vi "_io_viRead.vi"(8 "error in":errorcluster caption="error in (no error)", 9 "Allow Assure End with LF":bool=TRUE, 10 "Max bytes to read":u32=2048, 11 "VISA resource name":refnum<visa-resource-name>) -> (0 "error out":errorcluster, 1 "Read bytes count":u32, 2 "Read buffer":string, 3 "VISA resource name out":refnum<visa-resource-name>)   [LabVIEW 2020, in "Rohde&Schwarz RTx Oscilloscopes.lvlib" / "rsidr_core.lvlib"]
doc: "same as VISA viRead, but has an option to read the second time if the string was not ended with LF character"
uses:
  rsidr_core.lvlib
  type_AdditionalFlag_Bits.ctl
  type_Error_Codes.ctl
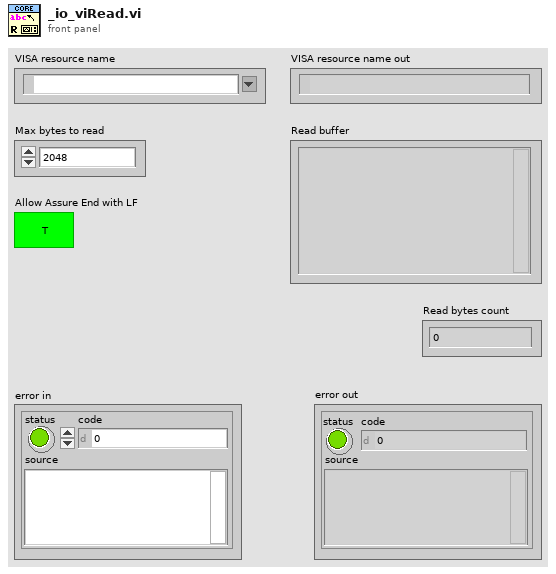
[diagram p1: front panel]
types:
  T1 = typedef "Rohde&Schwarz RTx Oscilloscopes.lvlib/rsidr_core.lvlib/type_AdditionalFlag_Bits.ctl" = enum16{"Send LF after Bin Block", "Junk read with io_clear_buffers.vi", "io_clear_buffers: viClear()", "io_clear_buffers: viFlush()", "<NotUsed1>", "Allow Dbl & Int Bin/Ascii read", "*OPC? in check_instrument_error.vi", "<NotUsed2>", "Smart Enum Matching", "Less Strict RepCaps check", "AssureResponseEndWithLF"}
  T2 = typedef "Rohde&Schwarz RTx Oscilloscopes.lvlib/rsidr_core.lvlib/type_Error_Codes.ctl" = enum16{"No_error", "VISA_err_ResourceNotFound", "VISA_err_Timeout", "VISA_warn_MoreDataAvailable", "RS_err_MissingCallback", "RS_err_InvalidAttribute", "RS_err_InvalidValue", "RS_err_UnknownResource", "RS_err_AlreadyInitialized", "RS_err_InstrumentStatus", "RS_err_BadRepCapName", "RS_err_TypesMismatch", "RS_err_ValueNotSupported", "RS_err_InvalidRngTable", "RS_err_IDqueryFail", "RS_err_UnexpResponse", "VISA_warn_ConfigNotLoaded", "RS_err_AttributeNotReadable", "RS_err_AttributeNotWritable", "RS_err_InstrumentType", "RS_err_InstrumentOption", "VISA_err_InvalidSize", "RS_err_ReliabilityIndicator", "VISA_warn_UnknownStatus", "VISA_warn_TermCharRead", "VISA_err_IO_error", "RS_err_FunctionNotSupported", "VISA_warn_QueueEmpty"}
  T3 = typedef "Rohde&Schwarz RTx Oscilloscopes.lvlib/rsidr_core.lvlib/type_Session_Data.ctl" = cluster{"IDN string":string, "Instrument FW":string, "Instr type":string, "Instr type for err. msg.":string, "Installed Options":string[], "Ignore Error Messages":string, "Logging params":variant, "OPC Timeout":i32, "VISA Timeout":i32, "STB Poll VISA Timeout":i32, "Additional Flags":i32, "Wait Before Read":i32, "Wait Before Write":i32, "Option String Flags":i32, "IO Segment Size":i64, "VISA Access Mode":T4, "Interface Type":T5, "OPC Wait Mode":T6, "Bin Float Number  Format":T7, "Bin Integer Number Format":T8, "Simulate":bool, "VXIcapable":bool, "Duplicate Session":bool, "Add LF to Write":bool, "Logging":bool, "Fast Sweep":bool, "Query Instrument Status":bool, "Check Range":bool, "Check Options":bool, "OPC-sync Attr Writes":bool, "OPC-sync Attr Queries":bool}
  T4 = typedef "Rohde&Schwarz RTx Oscilloscopes.lvlib/rsidr_core.lvlib/type_VisaAccessMode.ctl" = u16
  T5 = typedef "Rohde&Schwarz RTx Oscilloscopes.lvlib/rsidr_core.lvlib/type_InterfaceType.ctl" = enum16{"Unknown", "GPIB", "VXI", "GPIB_VXI", "ASRL", "PXI", "TCPIP", "USB", "SOCKET"}
  T6 = typedef "Rohde&Schwarz RTx Oscilloscopes.lvlib/rsidr_core.lvlib/type_OPC_Wait_Mode.ctl" = enum16{"STBpolling", "STBpollingSlow", "STBpollingSuperSlow", "ServiceRequest", "OPCquery"}
  T7 = typedef "Rohde&Schwarz RTx Oscilloscopes.lvlib/rsidr_core.lvlib/type_Binary_Float_Number_Format.ctl" = enum16{"Float_4_Bytes_Swapped", "Float_4_Bytes", "Double_8_Bytes_Swapped", "Double_8_Bytes"}
  T8 = typedef "Rohde&Schwarz RTx Oscilloscopes.lvlib/rsidr_core.lvlib/type_Binary_Integer_Number_Format.ctl" = enum16{"Int32_4_Bytes_Swapped", "Int32_4 Bytes", "Int16_2_Bytes_Swapped", "Int16_2_Bytes"}
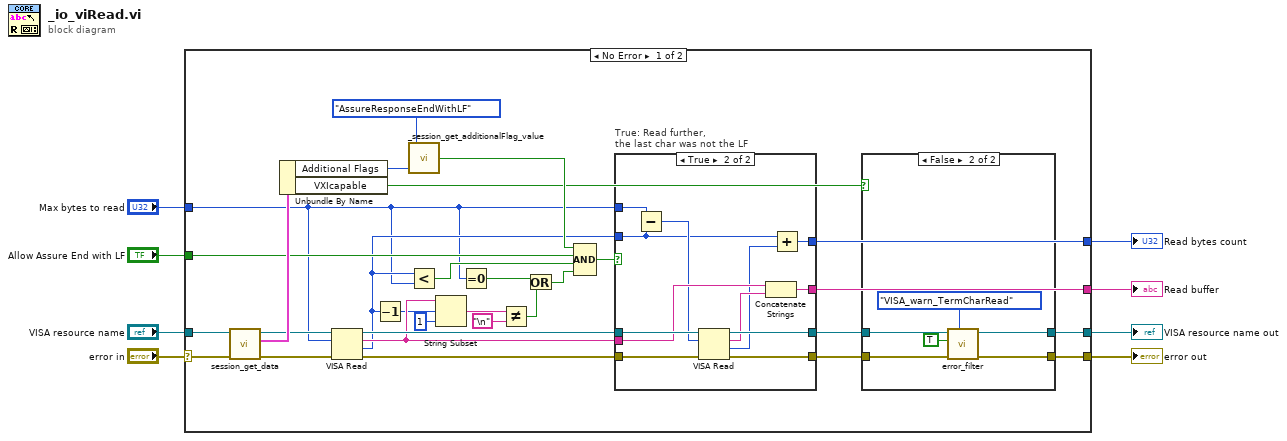
[diagram p0: block diagram]
diagram:
  n1 = case shown="No Error" "error in" {
    selector: "error in" -> [w35 w64]
    tunnel: [w38 w64] -> w7
    tunnel: "Max bytes to read" -> [w9 _]
    tunnel: "VISA resource name" -> [w34 w63]
    tunnel: [w37 w63] -> w6
    tunnel: [w24 _] -> w3
    tunnel: [w25 _] -> w2
    tunnel: "Allow Assure End with LF" -> [w27 _]
    frame No Error {
      n2 = call "session_get_data.vi"("error in"=w35, "VISA resource name"=w34) -> ("error out"=w33:errorcluster, "Session User Data out"=w36:T3, "VISA resource name out"=w32:refnum<visa-resource-name>)  [unwired: 6 in, 1 out]
      n3 = Unbundle By Name(w36) -> ("Additional Flags"=w31:i32, "VXIcapable"=w17:bool)
      n4 = VISA Read(VISA resource name=w32, byte count=w9, error in (no error)=w33) -> (VISA resource name out=w22:refnum<visa-resource-name>, read buffer=w16:string, return count=w15:u32, error out=w23:errorcluster)
      n5 = Decrement(x=w15) -> (x-1=w14:u32)
      n6 = call "_session_get_additionalFlag_value.vi"("AdditionalFlags value in"=w31, "AdditionalFlag bit"=type_AdditionalFlag_Bits."AssureResponseEndWithLF") -> ("AdditionalFlag bit value out"=w29:bool)  [unwired: 3 in]
      n7 = Less?(x=w15, y=w9) -> (x < y?=w28:bool)
      n8 = String Subset(string=w16, offset (0)=w14, length (rest)=1 ("length (rest)")) -> (substring=w12:string)
      n9 = Equal To 0?(x=w9) -> (x = 0?=w18:bool)
      n10 = Not Equal?(x=w12, y="\n" ("Line Feed Constant")) -> (x != y?=w10:bool)
      n11 = Or(x=w18, y=w10) -> (x .or. y?=w19:bool)
      n12 = Compound Arithmetic op=AND(w29, w27, w28, w19) -> (w26:bool)
      n13 = case "True: Read further,\nthe last char was not the LF" shown="True" w26 {
        tunnel: w16 -> [w42 w50]
        tunnel: [w42 w49] -> w25
        tunnel: w15 -> [w41 w43]
        tunnel: [w41 w46] -> w24
        tunnel: w23 -> [w40 w54]
        tunnel: w22 -> [w39 w53]
        tunnel: [w40 w52] -> w21
        tunnel: [w39 w51] -> w20
        tunnel: w9 -> [_ w44]
        frame False {
        }
        frame True {
          n14 = Subtract(x=w44, y=w43) -> (x-y=w45:u32)
          n15 = VISA Read(VISA resource name=w53, byte count=w45, error in (no error)=w54) -> (VISA resource name out=w51:refnum<visa-resource-name>, read buffer=w48:string, return count=w47:u32, error out=w52:errorcluster)
          n16 = Concatenate Strings(w50, w48) -> (w49:string)
          n17 = Add(x=w43, y=w47) -> (x+y=w46:u32)
        }
      }
      n18 = case shown="False" w17 {
        tunnel: w21 -> [w56 w60]
        tunnel: [w56 w58] -> w38
        tunnel: w20 -> [w55 w59]
        tunnel: [w55 w57] -> w37
        frame True {
        }
        frame False {
          n19 = call "error_filter.vi"("Error Enum in"=type_Error_Codes."VISA_warn_TermCharRead" ("Code to detect"), "error in"=w60, "Clear detected code (F)"=TRUE, "VISA resource name"=w59) -> ("error out"=w58:errorcluster, "VISA resource name out"=w57:refnum<visa-resource-name>)  [unwired: 5 in, 1 out]
        }
      }
    }
    frame Error {
    }
  }
  "VISA resource name out" <- w6
  "error out" <- w7
  "Read buffer" <- w2
  "Read bytes count" <- w3
